vi "OscilloscopeConfigurationFromCluster.vi"(8 "error in (no error)":errorcluster, 11 "output cluster":T1 {"vertical coupling" items=["AC", "DC", "Ground"]}) -> (0 "error out":errorcluster, 1 "active channel number string array":string[](array[string]), 2 "active channel number string list":string, 3 "IVI Refnum out":refnum<k15>)   [LabVIEW 2019]
uses:
  Controls/OscilloscopeBlockControl2.ctl
  <instrlib>/niScope/Controls/niScope vertical coupling.ctl
  <instrlib>/niScope/Configure/Trigger/niScope Configure Trigger Software.vi
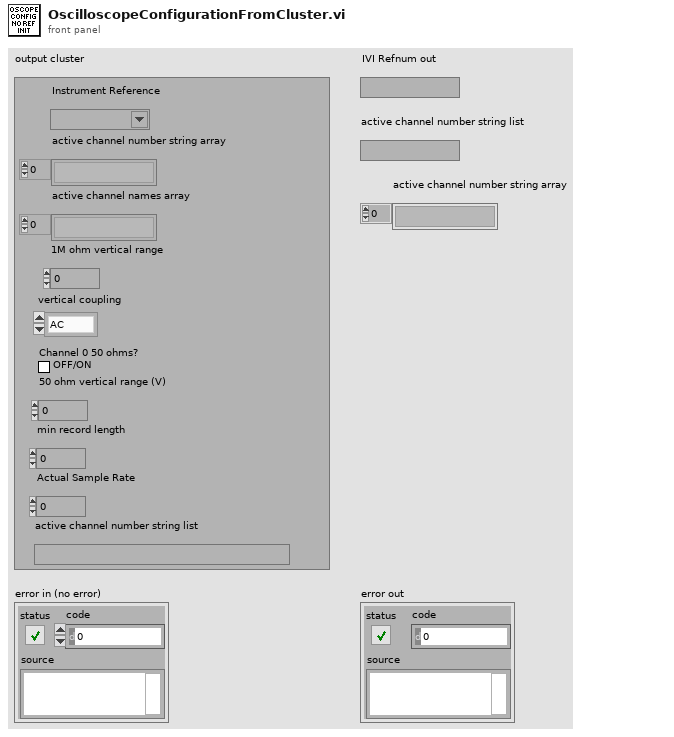
[diagram p1: front panel]
types:
  T1 = typedef "OscilloscopeBlockControl2.ctl" = cluster{"Instrument Reference":refnum<k15>, "active channel number string array":string[], "active channel names array":string[], "1M ohm vertical range":dbl, "vertical coupling":T2, "Channel 0 50 ohms?":bool, "50 ohm vertical range (V)":dbl, "min record length":i32, "Actual Sample Rate":dbl, "active channel number string list":string}
  T2 = typedef "niScope vertical coupling.ctl" = i32
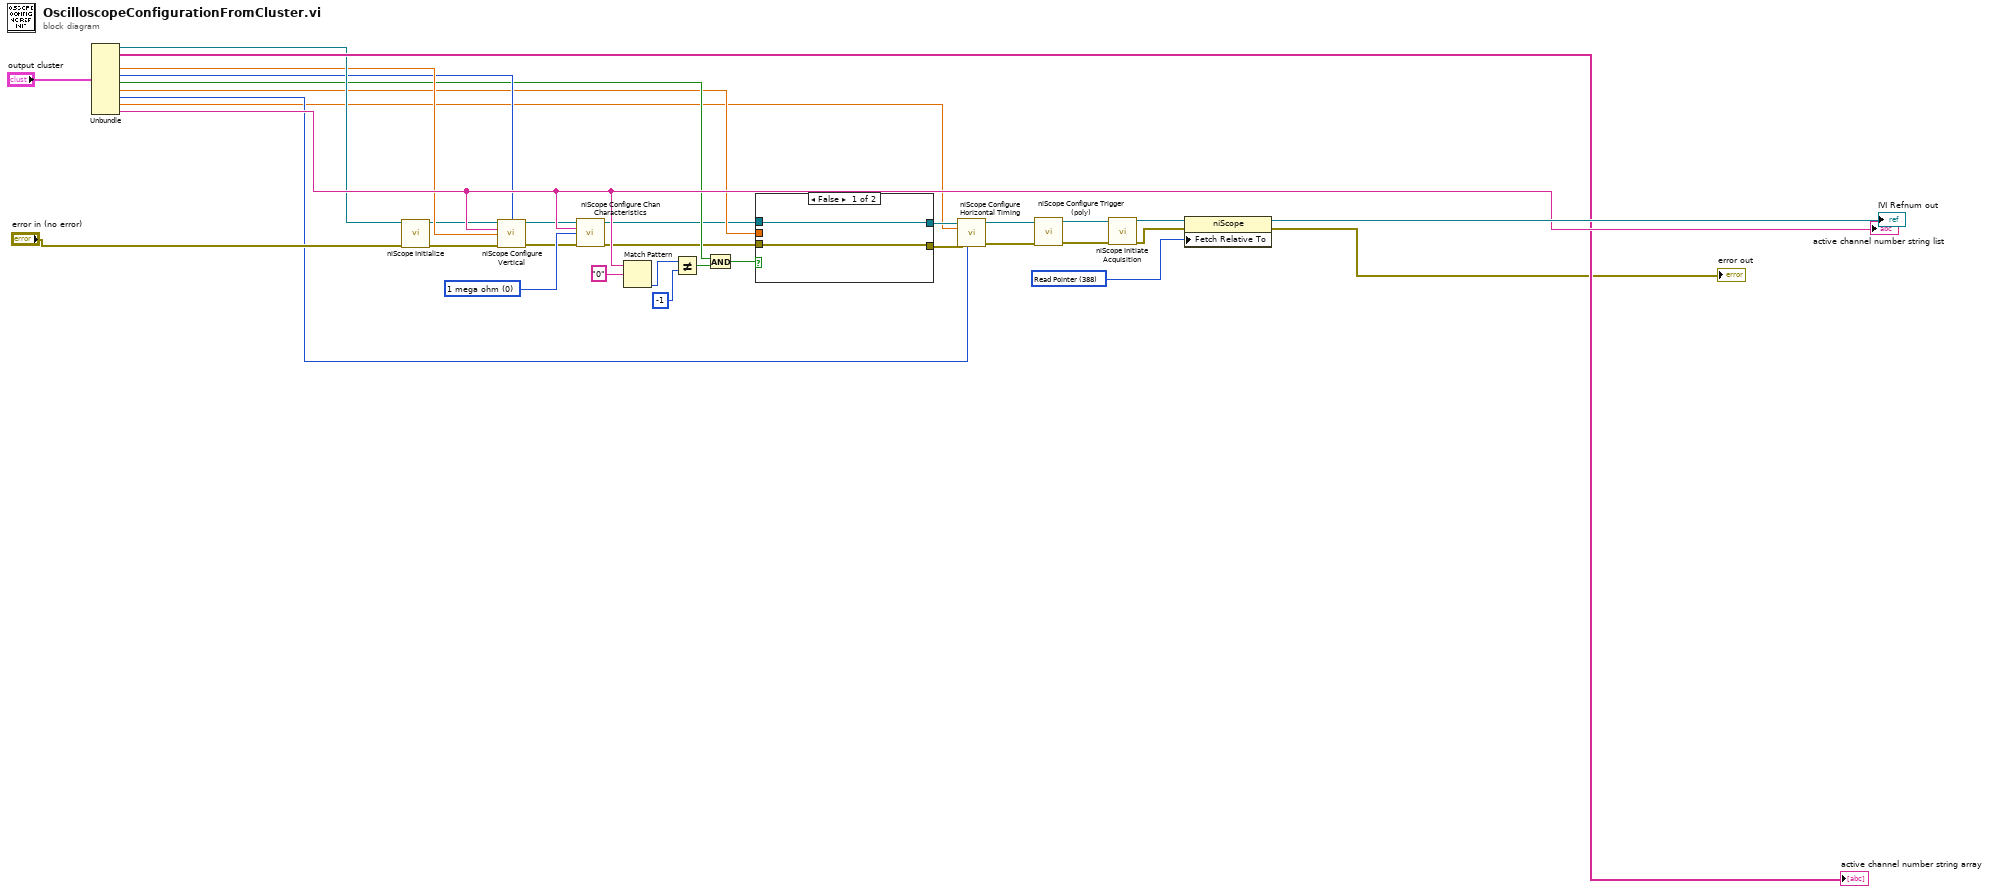
[diagram p0: block diagram]
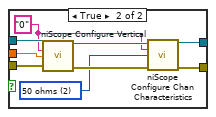
[diagram p2: hidden frame]
diagram:
  w12 = u32 0 items=["1 mega ohm"=0, "50 ohms"=2] ("input impedance")
  w7 = 388 items=["Start"=482, "Trigger"=483, "Pretrigger"=477, "Now"=481, "Read Pointer"=388] ("Fetch:Fetch Relative To")
  n1 = Unbundle("output cluster") -> ("Instrument Reference"=w30:refnum<k15>, "active channel number string array"=→"active channel number string array":string[], "1M ohm vertical range"=w29:dbl, "vertical coupling"=w28:T2, "Channel 0 50 ohms?"=w27:bool, "50 ohm vertical range (V)"=w24:dbl, "min record length"=w16:i32, "Actual Sample Rate"=w15:dbl, "active channel number string list"=w32:string)  [unwired: 1 out]
  "active channel number string list" <- w32
  n2 = call <instrlib>:"niScope Initialize.vi"("resource name"=w30, "error in"="error in (no error)") -> ("instrument handle"=w1:refnum<k15>, "error out"=w2:errorcluster)  [unwired: 12 in]
  n3 = call <instrlib>:"niScope Configure Vertical.vi"("instrument handle"=w1, "vertical coupling"=w28, "channels"=w32, "vertical range"=w29, "error in"=w2) -> ("instrument handle out"=w4:refnum<k15>, "error out"=w3:errorcluster)  [unwired: 9 in]
  n4 = call <instrlib>:"niScope Configure Chan Characteristics.vi"("instrument handle"=w4, "channels"=w32, "input impedance"=w12, "error in"=w3) -> ("instrument handle out"=w21:refnum<k15>, "error out"=w22:errorcluster)  [unwired: 10 in]
  n5 = Match Pattern(string=w32, regular expression="0") -> (offset past match=w18:i32)  [unwired: 1 in, 3 out]
  n6 = Not Equal?(x=w18, y=-1) -> (x != y?=w20:bool)
  n7 = And(x=w27, y=w20) -> (x .and. y?=w23:bool)
  n8 = case shown="False" w23 {
    tunnel: w21 -> [w36 w43]
    tunnel: w22 -> [w35 w42]
    tunnel: w24 -> [_ w40]
    tunnel: [w36 w38] -> w25
    tunnel: [w35 w37] -> w26
    frame False {
    }
    frame True {
      w39 = u32 2 items=["1 mega ohm"=0, "50 ohms"=2] ("input impedance")
      w41 = "0" ("channels")
      n9 = call <instrlib>:"niScope Configure Vertical.vi"("instrument handle"=w43, "channels"=w41, "vertical range"=w40, "error in"=w42) -> ("instrument handle out"=w45:refnum<k15>, "error out"=w44:errorcluster)  [unwired: 10 in]
      n10 = call <instrlib>:"niScope Configure Chan Characteristics.vi"("instrument handle"=w45, "channels"=w41, "input impedance"=w39, "error in"=w44) -> ("instrument handle out"=w38:refnum<k15>, "error out"=w37:errorcluster)  [unwired: 10 in]
    }
  }
  n11 = call <instrlib>:"niScope Configure Horizontal Timing.vi"("instrument handle"=w25, "min sample rate"=w15, "error in"=w26, "min record length"=w16) -> ("instrument handle out"=w6:refnum<k15>, "error out"=w5:errorcluster)  [unwired: 10 in]
  n12 = call-poly <instrlib>:"niScope Configure Trigger (poly).vi"("instrument handle"=w6, "error in"=w5) -> ("instrument handle out"=w8:refnum<k15>, "error out"=w9:errorcluster)  [unwired: 12 in]
  n13 = call <instrlib>:"niScope Initiate Acquisition.vi"("instrument handle"=w8, "error in"=w9) -> ("instrument handle out"=w11:refnum<k15>, "error out"=w10:errorcluster)  [unwired: 12 in]
  n14 = property class="niScope"(reference=w11, error in=w10, "Fetch Relative To"=w7) -> (reference out=→"IVI Refnum out":refnum<k15>, error out=→"error out":errorcluster)
